vi "XControl with User Events Method.vi"(0 "Display State In":T1, 9 "Container State":T2, 11 "error in (no error)":errorcluster) -> (4 "Display State Out":T1, 6 "User Event Time":refnum<user-event>, 15 "error out":errorcluster)   [LabVIEW 2009, in "XControlUserEvents.xctl"]
doc: "Demonstration of an XControl.\n\nAAL 9/09"
uses:
  XControlUserEvents.xctl
  <vilib>/_xctls/Container State.ctl
  Abilities/XControl with User Events State.ctl
  <vilib>/_xctls/XControlSupport.lvlib
panel:
  # "Add Controls & Indicators that form the parameters of the method here. Hook them to the connector pane. Do not delete the controls & indicators that are already hooked to the connector pane.\n \nTo setup the parameters  for this method, right click on this item in the Project Tree & select \"Configure Method...\"."
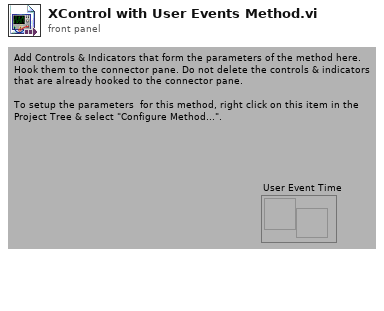
[diagram p1: front panel]
types:
  T1 = typedef "XControlUserEvents.xctl/XControl with User Events State.ctl" = cluster{"Numeric":dbl, "user event":refnum<user-event>, "String":string}
  T2 = typedef "XControlSupport.lvlib/Container State.ctl" = cluster{"Indicator?":bool, "Run Mode?":bool, " Refnum":refnum<vi>}
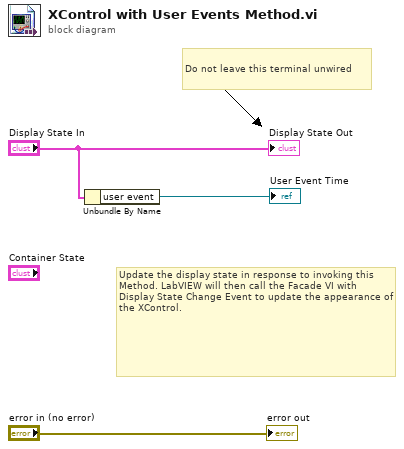
[diagram p0: block diagram]
diagram:
  # "Do not leave this terminal unwired"
  # "Update the display state in response to invoking this Method. LabVIEW will then call the Facade VI with Display State Change Event to update the appearance of the XControl."
  n1 = Unbundle By Name("Display State In") -> ("user event"=→"User Event Time":refnum<user-event>)
  "Display State Out" <- "Display State In"
  "error out" <- "error in (no error)"
